vi "ANAL_SurfaceGet.vi"(6 "Sweep Range":cluster{"Numeric":i32, "Numeric":i32}, 9 "Target Set Points":i32[](array[numeric]), 11 "Run Data Cluster":T1 {"Temperature B" scale=0.0..100.0; "Temperature A" scale=0.0..100.0}) -> (2 "Normalised Surface":dbl[][](array[numeric]))   [LabVIEW 2021]
uses:
  DAT_Cluster.ctl
  81de8623-b3e4-400a-9ecc-59d5fbcc5fd3.vi
  81de8623-b3e4-400a-9ecc-59d5fbcc5fd3.vi/d4db2432-cc9c-482c-8957-dac855435ef6.vi
  81de8623-b3e4-400a-9ecc-59d5fbcc5fd3.vi/86fbf154-bd7b-49a2-8ab2-a837b2a95f24.vi
  81de8623-b3e4-400a-9ecc-59d5fbcc5fd3.vi/3b95b01e-1ec2-4565-bcd9-7606a5281010.vi
  81de8623-b3e4-400a-9ecc-59d5fbcc5fd3.vi/96a08935-737a-44b2-979c-a81d56408f7e.vi
  81de8623-b3e4-400a-9ecc-59d5fbcc5fd3.vi/d4db2432-cc9c-482c-8957-dac855435ef6.vi/6eaecd13-6e48-4772-a921-b51ebdf84d88.vi
  81de8623-b3e4-400a-9ecc-59d5fbcc5fd3.vi/d4db2432-cc9c-482c-8957-dac855435ef6.vi/d2d5f2b7-06f4-47f6-971c-049c3fdbb653.vi
  81de8623-b3e4-400a-9ecc-59d5fbcc5fd3.vi/3b95b01e-1ec2-4565-bcd9-7606a5281010.vi/6eaecd13-6e48-4772-a921-b51ebdf84d88.vi
  81de8623-b3e4-400a-9ecc-59d5fbcc5fd3.vi/3b95b01e-1ec2-4565-bcd9-7606a5281010.vi/d2d5f2b7-06f4-47f6-971c-049c3fdbb653.vi
  81de8623-b3e4-400a-9ecc-59d5fbcc5fd3.vi/96a08935-737a-44b2-979c-a81d56408f7e.vi/6eaecd13-6e48-4772-a921-b51ebdf84d88.vi
  81de8623-b3e4-400a-9ecc-59d5fbcc5fd3.vi/96a08935-737a-44b2-979c-a81d56408f7e.vi/d2d5f2b7-06f4-47f6-971c-049c3fdbb653.vi
  <vilib>/Comparison/Less/Less Functor/Less Functor.lvclass
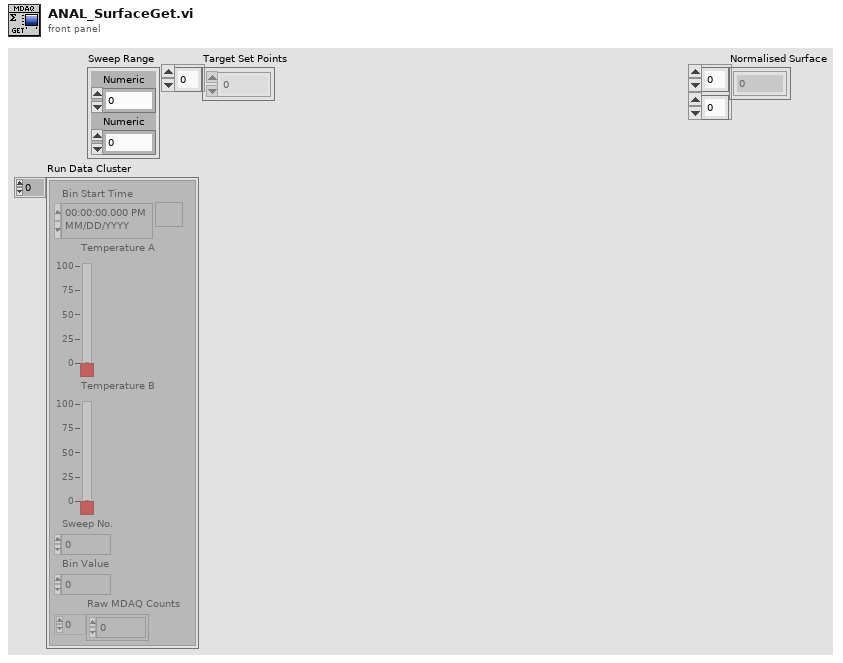
[diagram p1: front panel]
types:
  T1 = typedef "DAT_Cluster.ctl" = cluster{"Bin Start Time":timestamp, "Temperature A":dbl, "Temperature B":dbl, "Sweep No.":i32, "Bin Value":i32, "Raw MDAQ Counts":i32[]}[]
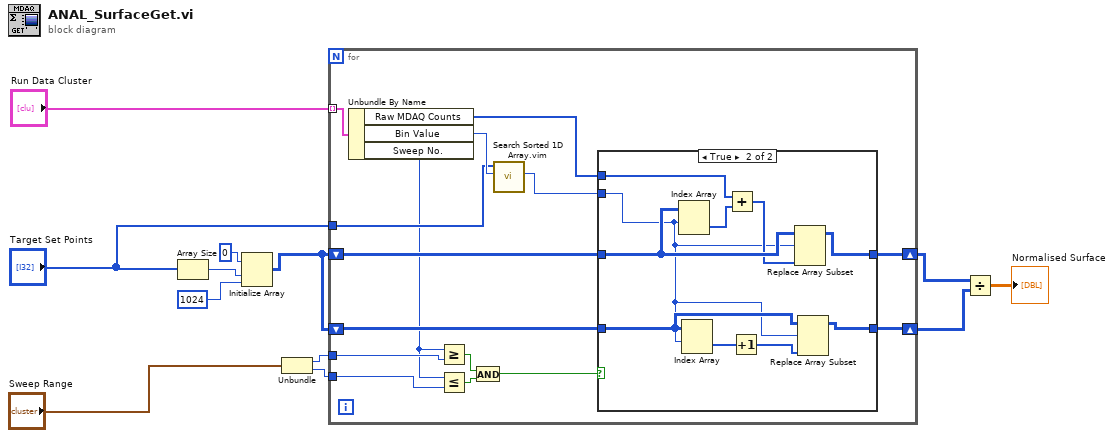
[diagram p0: block diagram]
diagram:
  n1 = Array Size(array="Target Set Points") -> (size(s)=w11:i32)
  n2 = Initialize Array(0 ("element"), w11, 1024 ("dimension size")) -> (w6:i32[][])
  n3 = Unbundle("Sweep Range") -> ("Numeric"=w5:i32, "Numeric"=w4:i32)
  n4 = for {
    tunnel: "Run Data Cluster" -> [w27] mode=indexing
    shift-right: [w23] -> w3
    shift-left: w6 -> [w24]
    tunnel: "Target Set Points" -> [w25]
    shift-right: [w19] -> w2
    shift-left: w6 -> [w20]
    tunnel: w5 -> [w18]
    tunnel: w4 -> [w16]
    n5 = Unbundle By Name(w27) -> ("Raw MDAQ Counts"=w21:i32[], "Bin Value"=w26:i32, "Sweep No."=w17:i32)
    n6 = Greater Or Equal?(x=w17, y=w18) -> (x >= y?=w15:bool)
    n7 = Less Or Equal?(x=w17, y=w16) -> (x <= y?=w14:bool)
    n8 = And(x=w15, y=w14) -> (x .and. y?=w13:bool)
    n9 = call "Search Sorted 1D Array.vim"("element"=w26, "sorted 1D array"=w25) -> ("nearest index"=w22:i32)  [unwired: 8 in, 1 out]
    n10 = case shown="True" w13 {
      tunnel: w24 -> [w29 w37]
      tunnel: [w29 w35] -> w23
      tunnel: w22 -> [_ w32]
      tunnel: w21 -> [_ w39]
      tunnel: w20 -> [w28 w33]
      tunnel: [w28 w30] -> w19
      frame False {
      }
      frame True {
        n11 = Index Array(array=w37, index (row)=w32) -> (element=w38:i32[])  [unwired: 1 in]
        n12 = Index Array(array=w33, index (row)=w32) -> (element=w34:i32[])  [unwired: 1 in]
        n13 = Add(x=w39, y=w38) -> (x+y=w36:i32[])
        n14 = Increment(x=w34) -> (x+1=w31:i32[])
        n15 = Replace Array Subset(array=w37, new element=w36, index (row)=w32) -> (w35:i32[][])  [unwired: 1 in]
        n16 = Replace Array Subset(array=w33, new element=w31, index (row)=w32) -> (w30:i32[][])  [unwired: 1 in]
      }
    }
  }
  n17 = Divide(x=w3, y=w2) -> (x/y=→"Normalised Surface":dbl[][])
